vi "UI Initialize.vi"(8 "error in (no error)":errorcluster, 11 "UI ActorTop in":refnum<class "Model_AMC.lvclass">) -> (0 "error out":errorcluster, 3 "UI ActorTop out":refnum<class "Model_AMC.lvclass">)   [LabVIEW 2021, in "Model_AMC.lvclass"]
doc: "UI: Initialize\n2015-03-18 16:27:22\n蒋松\njiangsong@outlook.com"
uses:
  Model_AMC.lvclass
  Model_AMC.lvclass/Model_AMC.ctl
  <vilib>/ActorFramework/Actor/Actor.lvclass
  <userlib>/John_Lib/AbstractActorTemplate/AbstractActorTemplate/UIActorTop.lvclass
  C:/Program Files (x86)/National Instruments/LabVIEW 2021/user.lib/John_Lib/AbstractActorTemplate/AbstractActorTemplate/UIActorTop.lvclass
  C:/Program Files (x86)/National Instruments/LabVIEW 2021/vi.lib/ActorFramework/Actor/Actor.lvclass
  C:/Program Files (x86)/National Instruments/LabVIEW 2021/project/Create Actor from Template/_Model_AMC/Model_AMC.lvclass
  C:/Program Files (x86)/National Instruments/LabVIEW 2021/user.lib/John_Lib/Interfaces/InsertUpDownSubPanel/InsertUpDownSubPanel.lvclass
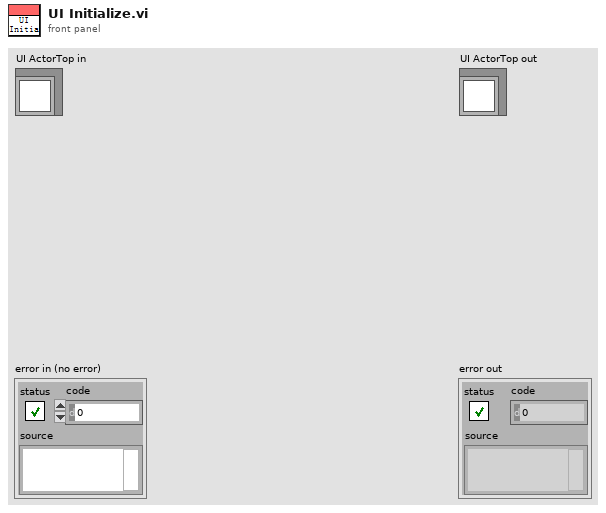
[diagram p1: front panel]
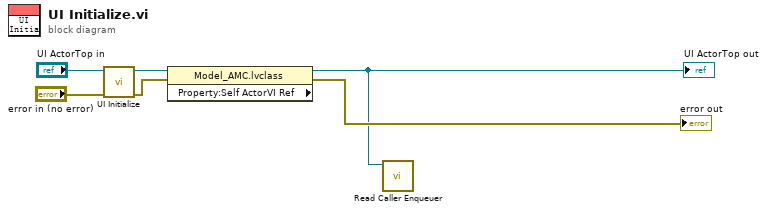
[diagram p0: block diagram]
diagram:
  n1 = call-parent "UI Initialize.vi"("error in (no error)"="error in (no error)", "UI ActorTop in"="UI ActorTop in") -> ("error out"=w3:errorcluster, "UI ActorTop out"=w5:refnum<class "Model_AMC.lvclass">)  [unwired: 8 in]
  n2 = property class="Model_AMC.lvclass" props=["Property:Self ActorVI Ref"](reference=w5, error in=w3) -> (reference out=w1:refnum<class "Model_AMC.lvclass">, error out=→"error out":errorcluster)  [unwired: 1 out]
  "UI ActorTop out" <- w1
  n3 = call <vilib>:"Read Caller Enqueuer.vi"("Actor"=w1) -> ()  [unwired: 10 in, 1 out]
